vi "Manual.vi"(8 "error in (no error)":errorcluster, 10 "Shutters":T1, 11 "Container in":refnum<class "Container.lvclass">) -> (0 "error out":errorcluster, 3 "Container out":refnum<class "Container.lvclass">)   [LabVIEW 2016, in "Container.lvclass"]
uses:
  Container.lvclass
  Controls/Shutters.ctl
  Controls/Shutter Data.ctl
  Controls/Shutter States.ctl
  Container.lvclass/Container.ctl
  Sci/SciShutt.lvclass
  LFCSim/LFCSimShutt.lvclass
  ExtFlat/ExtFlatShutt.lvclass
  SimFlat/SimFlatShutt.lvclass
  Solar/SolarShutt.lvclass
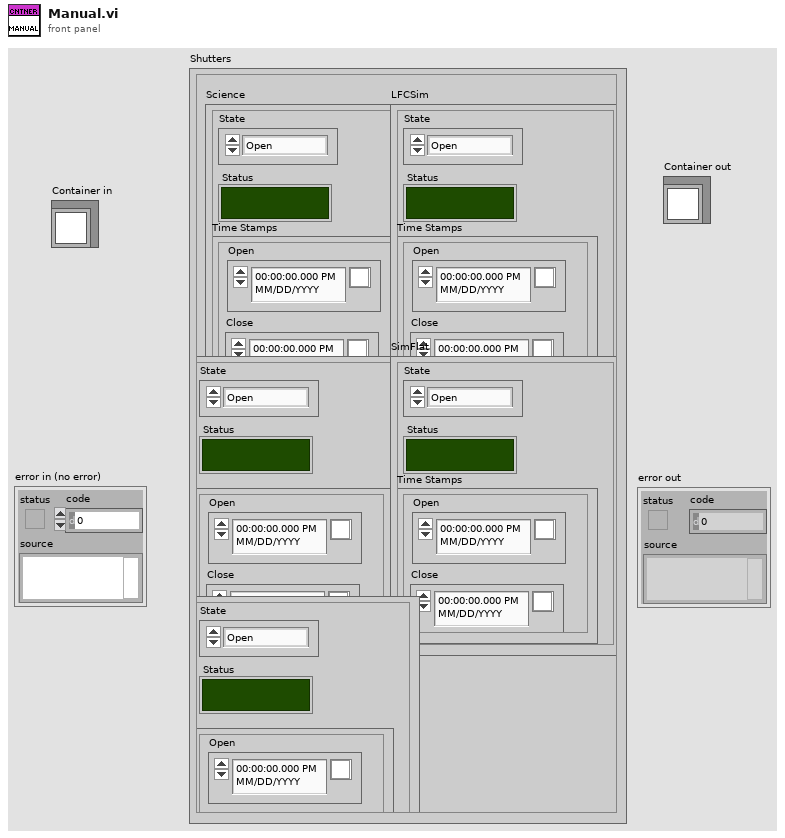
[diagram p1: front panel]
types:
  T1 = typedef "Shutters.ctl" = cluster{"Science":T2, "LFCSim":T2, "ExtendFlat":T2, "SimFlat":T2, "Solar":T2}
  T2 = typedef "Shutter Data.ctl" = cluster{"Status":bool, "State":T3, "Time Stamps":cluster{"Open":timestamp, "Close":timestamp}}
  T3 = typedef "Shutter States.ctl" = enum16{"Open", "Close", "Wait", "Off", "Arm", "Idle"}
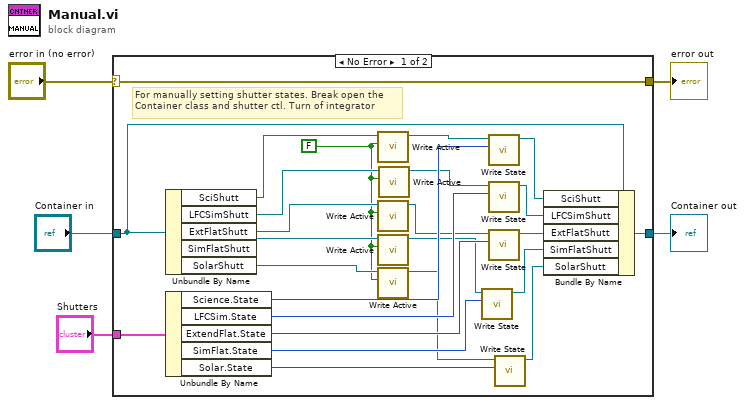
[diagram p0: block diagram]
diagram:
  n1 = case shown="No Error" "error in (no error)" {
    selector: "error in (no error)" -> [w21 w32]
    tunnel: [w21 w32] -> w4
    tunnel: [w30 w31] -> w2
    tunnel: "Container in" -> [w28 w31]
    tunnel: "Shutters" -> [w29 _]
    frame No Error {
      w6 = FALSE ("Active")
      # "For manually setting shutter states. Break open the\nContainer class and shutter ctl. Turn of integrator"
      n2 = Unbundle By Name(w28) -> ("SciShutt"=w17:refnum<class "SciShutt.lvclass">, "LFCSimShutt"=w15:refnum<class "LFCSimShutt.lvclass">, "ExtFlatShutt"=w13:refnum<class "ExtFlatShutt.lvclass">, "SimFlatShutt"=w10:refnum<class "SimFlatShutt.lvclass">, "SolarShutt"=w9:refnum<class "SolarShutt.lvclass">)
      n3 = Unbundle By Name(w29) -> ("Science.State"=w19:T3, "LFCSim.State"=w20:T3, "ExtendFlat.State"=w26:T3, "SimFlat.State"=w24:T3, "Solar.State"=w23:T3)
      n4 = call-dynamic "Write Active.vi"("Active"=w6, "Integrator in"=w17) -> ("Integrator out"=w16:refnum<class "SciShutt.lvclass">)  [unwired: 8 in, 1 out]
      n5 = call-dynamic "Write Active.vi"("Active"=w6, "Integrator in"=w13) -> ("Integrator out"=w12:refnum<class "ExtFlatShutt.lvclass">)  [unwired: 8 in, 1 out]
      n6 = call-dynamic "Write Active.vi"("Active"=w6, "Integrator in"=w10) -> ("Integrator out"=w11:refnum<class "SimFlatShutt.lvclass">)  [unwired: 8 in, 1 out]
      n7 = call-dynamic "Write Active.vi"("Active"=w6, "Integrator in"=w9) -> ("Integrator out"=w8:refnum<class "SolarShutt.lvclass">)  [unwired: 8 in, 1 out]
      n8 = call-dynamic "Write Active.vi"("Active"=w6, "Integrator in"=w15) -> ("Integrator out"=w14:refnum<class "LFCSimShutt.lvclass">)  [unwired: 8 in, 1 out]
      n9 = call-dynamic "Write State.vi"("Set"=w24, "Shutter in"=w11) -> ("Shutter out"=w7:refnum<class "SimFlatShutt.lvclass">)  [unwired: 8 in, 1 out]
      n10 = call-dynamic "Write State.vi"("Set"=w19, "Shutter in"=w16) -> ("Shutter out"=w18:refnum<class "SciShutt.lvclass">)  [unwired: 8 in, 1 out]
      n11 = call-dynamic "Write State.vi"("Set"=w20, "Shutter in"=w14) -> ("Shutter out"=w27:refnum<class "LFCSimShutt.lvclass">)  [unwired: 8 in, 1 out]
      n12 = call-dynamic "Write State.vi"("Set"=w26, "Shutter in"=w12) -> ("Shutter out"=w25:refnum<class "ExtFlatShutt.lvclass">)  [unwired: 8 in, 1 out]
      n13 = call-dynamic "Write State.vi"("Set"=w23, "Shutter in"=w8) -> ("Shutter out"=w22:refnum<class "SolarShutt.lvclass">)  [unwired: 8 in, 1 out]
      n14 = Bundle By Name(cluster=w28, "SciShutt"=w18, "LFCSimShutt"=w27, "ExtFlatShutt"=w25, "SimFlatShutt"=w7, "SolarShutt"=w22) -> (w30:refnum<class "Container.lvclass">)
    }
    frame Error {
    }
  }
  "error out" <- w4
  "Container out" <- w2
